vi "Send_Get_8Bits.vi"(8 "error in (no error)":errorcluster, 10 "Channel":u8, 11 "Serial Device in":refnum<class "Serial Device.lvclass">) -> (0 "error out":errorcluster, 2 "Response":string, 3 "Serial Device out":refnum<class "Serial Device.lvclass">)   [LabVIEW 2019, in "Serial Device.lvclass"]
uses:
  Serial Device.lvclass
  Serial Device.lvclass/Serial Device.ctl
  0713ec9a-b44c-44ab-a500-c5f2b92f772c.vi
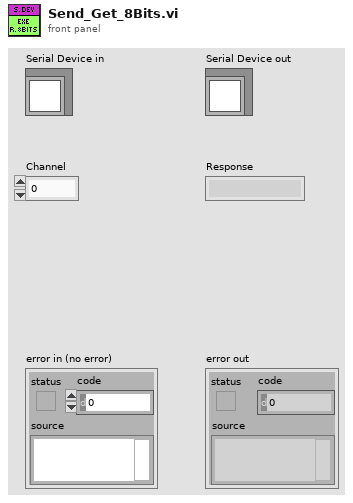
[diagram p1: front panel]
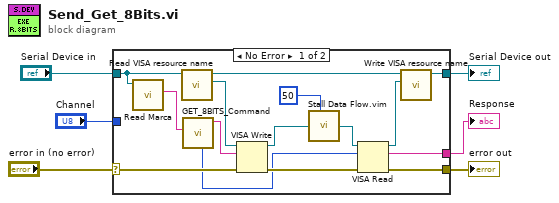
[diagram p0: block diagram]
diagram:
  n1 = case shown="No Error" "error in (no error)" {
    selector: "error in (no error)" -> [w19 w23]
    tunnel: [w15 w23] -> w5
    tunnel: [w11 w22] -> w3
    tunnel: "Serial Device in" -> [w21 w22]
    tunnel: "Channel" -> [_ _]
    tunnel: [w10 _] -> w1
    frame No Error {
      n2 = call "Read Marca.vi"("Serial Device in"=w21) -> ("Marca"=w9:string)  [unwired: 8 in, 2 out]
      n3 = call "Read VISA resource name.vi"("Serial Device in"=w21) -> ("VISA resource name"=w20:refnum<visa-resource-name>, "Serial Device out"=w12:refnum<class "Serial Device.lvclass">)  [unwired: 8 in, 1 out]
      n4 = call "GET_8BITS_Command.vi"("Marca"=w9) -> ("Command"=w7:string, "Bytes Expected"=w8:u32)  [unwired: 7 in, 2 out]
      n5 = VISA Write(VISA resource name=w20, write buffer=w7, error in (no error)=w19) -> (VISA resource name out=w18:refnum<visa-resource-name>, error out=w16:errorcluster)  [unwired: 1 out]
      n6 = call "Stall Data Flow.vim"("value in"=w18, "milliseconds to wait"=u32 50) -> ("value out"=w17:refnum<visa-resource-name>)  [unwired: 1 out]
      n7 = VISA Read(VISA resource name=w17, byte count=w8, error in (no error)=w16) -> (VISA resource name out=w13:refnum<visa-resource-name>, read buffer=w10:string, error out=w15:errorcluster)  [unwired: 1 out]
      n8 = call "Write VISA resource name.vi"("VISA resource name"=w13, "Serial Device in"=w12) -> ("Serial Device out"=w11:refnum<class "Serial Device.lvclass">)  [unwired: 8 in, 1 out]
    }
    frame Error {
    }
  }
  "error out" <- w5
  "Serial Device out" <- w3
  "Response" <- w1
